vi "DHE_set_artifpattern.vi"(0 "fd":i32, 7 "artifpattern":string, 11 "error in (no error)":errorcluster) -> (4 "fd out":i32, 8 "return value":i32, 15 "error out":errorcluster)   [LabVIEW 2016]
doc: "This VI opens (Flag=1) or closes (Flag=0) the instrument shutter."
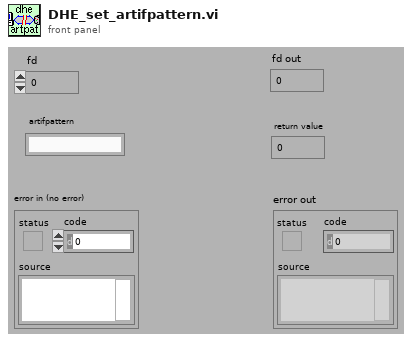
[diagram p1: front panel]
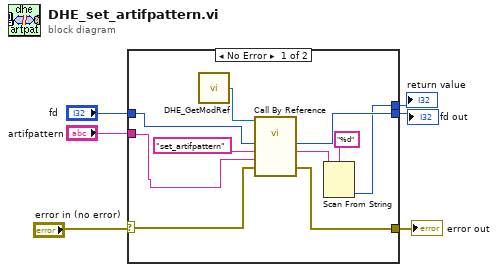
[diagram p0: block diagram]
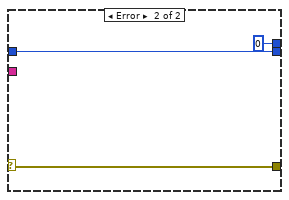
[diagram p2: hidden frame]
diagram:
  n1 = case shown="No Error" "error in (no error)" {
    selector: "error in (no error)" -> [w14 w17]
    tunnel: "fd" -> [w12 w19]
    tunnel: [w8 0] -> w5
    tunnel: [w13 w17] -> w4
    tunnel: "artifpattern" -> [w7 _]
    tunnel: [w11 w19] -> w2
    frame No Error {
      n2 = call "DHE_GetModRef.vi"() -> ("DHE_ModRef"=w16:refnum<vi>)  [unwired: 9 out]
      n3 = call-by-ref "?"(reference=w16, "error in (no error)"=w14, "arguments"=w7, "function"="set_artifpattern", "fd in"=w12) -> ("error out"=w13:errorcluster, "str result"=w10:string, "fd out"=w11:i32)  [unwired: 5 in, 3 out]
      n4 = Scan From String(format string="%d", input string=w10) -> (output 1=w8:i32)  [unwired: 2 in, 4 out]
    }
    frame Error {
    }
  }
  "error out" <- w4
  "return value" <- w5
  "fd out" <- w2
